vi "BeeHarmonicRadar.vi"(1 "Sampling Period":u32=10, 2 "Encoder Velocity Configuration":T1={"Right Encoder Rate to Velocity"=1.0, "Left Encoder Rate to Velocity"=1.0}, 3 "Reckoned Position FIFO Name":string="Position", 4 "Yaw RT FIFO":string="Yaw", 5 "Initial Values":T7, 6 "Encoder Dev Refs":T6={"RightEncoderDevRef"={"DevStatus"={"status"=FALSE, "code"=0, "source"=""}, "EncoderIndex"=enum."Invalid", "CounterIndex"=enum."Invalid", "DistancePerCount"=1.0, "Decoding Type"=enum."4x"}, "LeftEncoderDevRef"={"DevStatus"={"status"=FALSE, "code"=0, "source"=""}, "EncoderIndex"=enum."Invalid", "CounterIndex"=enum."Invalid", "DistancePerCount"=1.0, "Decoding Type"=enum."4x"}}) -> ()   [LabVIEW 2016]
uses:
  <vilib>/Rock Robotics/WPI/Encoder/WPI_EncoderDevRef.ctl
  <vilib>/Rock Robotics/SystemInterfaces/Encoder/FPGA_EncoderIdx.ctl
  <vilib>/Rock Robotics/SystemInterfaces/Counter/FPGA_CounterCtrSystemIndex.ctl
  <vilib>/Rock Robotics/WPI/Encoder/WPI_EncoderType.ctl
  <vilib>/Platform/TimedLoop/XDataNode/timing_clust.ctl
  <vilib>/Platform/TimedLoop/XDataNode/nitl_modes.ctl
  <vilib>/Platform/TimedLoop/XDataNode/wakeup.ctl
  <vilib>/platform/TimedLoop/XDataNode/XDataNode.xnode
  <vilib>/Platform/TimedLoop/XDataNode/XDNodeRunTimeDep.lvlib
panel:
  out "Y Trap + Gyro":dbl
  out "X Trap + Gyro":dbl
  in  "Reset":bool
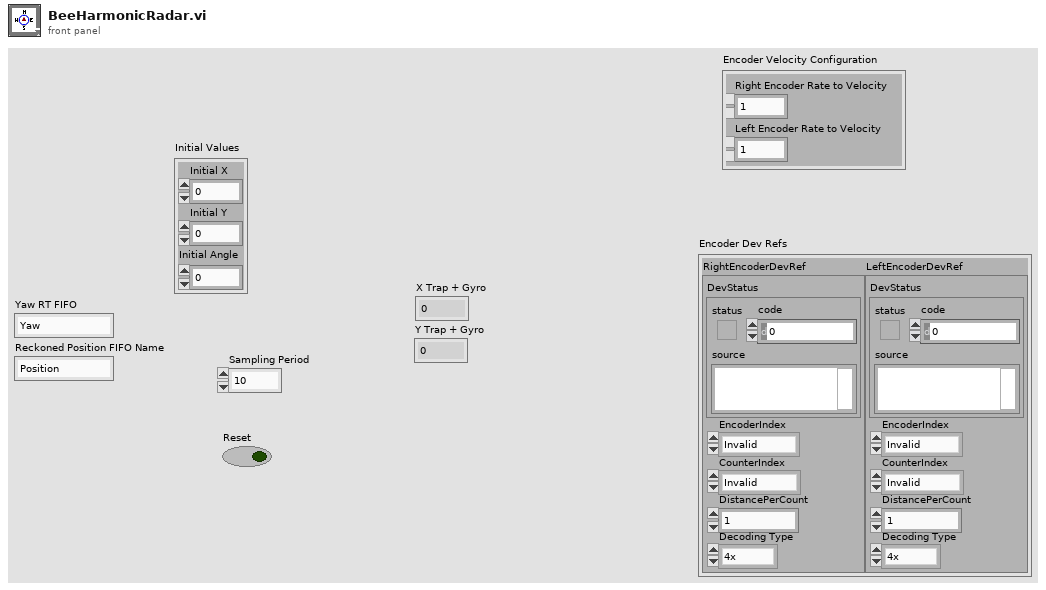
[diagram p1: front panel]
types:
  T1 = cluster{"Right Encoder Rate to Velocity":dbl, "Left Encoder Rate to Velocity":dbl}
  T2 = typedef "WPI_EncoderDevRef.ctl" = cluster{"DevStatus":errorcluster, "EncoderIndex":T3, "CounterIndex":T4, "DistancePerCount":dbl, "Decoding Type":T5}
  T3 = typedef "FPGA_EncoderIdx.ctl" = enum8{"Enc 0", "Enc 1", "Enc 2", "Enc 3", "Enc 4", "Enc 5", "Enc 6", "Enc 7", "Invalid"}
  T4 = typedef "FPGA_CounterCtrSystemIndex.ctl" = enum8{"Ctr 0", "Ctr 1", "Ctr 2", "Ctr 3", "Ctr 4", "Ctr 5", "Ctr 6", "Ctr 7", "Invalid"}
  T5 = typedef "WPI_EncoderType.ctl" = enum16{"1x", "2x", "4x"}
  T6 = cluster{"RightEncoderDevRef":T2, "LeftEncoderDevRef":T2}
  T7 = cluster{"Initial X":dbl, "Initial Y":dbl, "Initial Angle":dbl}
  T8 = typedef "XDNodeRunTimeDep.lvlib/timing_clust.ctl" = cluster{"Expected End [f-1]":u64, "Actual End [f-1]":u64, "Finished Late? [f-1]":bool, "Expected End [i-1]":u64, "Actual End [i-1]":u64, "Finished Late? [i-1]":bool, "Expected Start [i]":u64, "Actual Start [i]":u64, "Expected Start [f]":u64, "Actual Start [f]":u64, "Source Name":string, "Structure Name":string, "Period":i64, "Deadline":i64, "Offset":i64, "Start":i64, "Priority":i32, "Timeout":i32, "Mode":T9, "Wakeup Reason":T10, "Error":errorcluster, "Source Type":string, "Secondary Source Type":string, "Global End Time":u64, "Global Start Time":u64, "Frame Duration":u64, "Iteration Duration":u64, "Assigned CPU":i32, "I/O Scan Engine Mode":u32}
  T9 = typedef "XDNodeRunTimeDep.lvlib/nitl_modes.ctl" = enum32{"No Change", "Process missed periods, maintain original phase", "Discard missed periods, maintain original phase", "Process missed periods, ignore original phase", "Discard missed periods, ignore original phase"}
  T10 = typedef "XDNodeRunTimeDep.lvlib/wakeup.ctl" = enum32{"Normal", "Aborted", "Asynchronous wakeup", "Timing source error", "Timed loop error", "Timeout"}
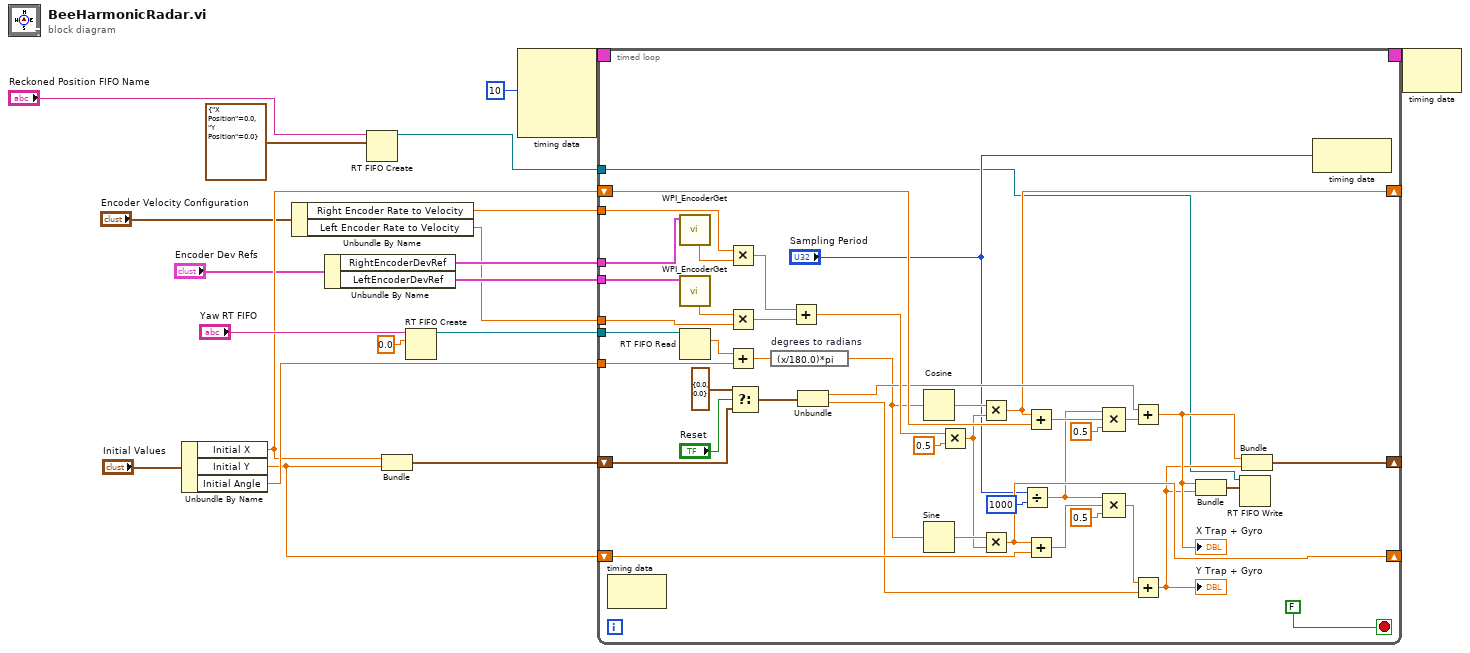
[diagram p0: block diagram]
diagram:
  n1 = Unbundle By Name("Initial Values") -> ("Initial X"=w7:dbl, "Initial Y"=w8:dbl, "Initial Angle"=w9:dbl)
  n2 = Unbundle By Name("Encoder Velocity Configuration") -> ("Right Encoder Rate to Velocity"=w2:dbl, "Left Encoder Rate to Velocity"=w1:dbl)
  n3 = Unbundle By Name("Encoder Dev Refs") -> ("RightEncoderDevRef"=w5:T2, "LeftEncoderDevRef"=w4:T2)
  n4 = RT FIFO Create(0:"Reckoned Position FIFO Name", 1:cluster{"X Position":dbl, "Y Position":dbl} {"X Position"=0.0, "Y Position"=0.0}) -> (8:w11:refnum<k33>)  [unwired: 6 in, 2 out]
  n5 = Bundle("Initial X"=w7, "Initial Y"=w8) -> (w20:cluster{"Initial X":dbl, "Initial Y":dbl})  [unwired: 1 in]
  n6 = RT FIFO Create(0:"Yaw RT FIFO", 1:0.0) -> (8:w16:refnum<k33>)  [unwired: 6 in, 2 out]
  n7 = node-c288(i64 10 ("Period")) -> (w19:T8)  [unwired: 3 in]
  n8 = timed-loop {
    tunnel: w9 -> [w62]
    shift-right: [w46] -> _
    shift-left: w8 -> [w60]
    shift-right: [w43] -> _
    shift-left: w7 -> [w59]
    shift-right: [w50] -> _
    shift-left: w20 -> [w32]
    timing: w19 -> [_]
    timing-out: [_] -> w18
    tunnel: w4 -> [w42]
    tunnel: w5 -> [w41]
    tunnel: w16 -> [w28]
    tunnel: w11 -> [w23]
    tunnel: w2 -> [w22]
    tunnel: w1 -> [w21]
    stop <- FALSE stop-if-true
    n9 = node-c288() -> ()  [unwired: 1 in, 1 out]
    n10 = call <vilib>:"WPI_EncoderGet.vi"("EncoderDevRef"=w41) -> ("Rate"=w30:dbl)  [unwired: 5 in, 5 out]
    n11 = call <vilib>:"WPI_EncoderGet.vi"("EncoderDevRef"=w42) -> ("Rate"=w29:dbl)  [unwired: 5 in, 5 out]
    n12 = RT FIFO Read(0:w28) -> (9:w27:dbl)  [unwired: 3 in, 4 out]
    n13 = Multiply(x=w22, y=w30) -> (x*y=w40:dbl)
    n14 = Multiply(x=w29, y=w21) -> (x*y=w39:dbl)
    n15 = Add(x=w27, y=w62) -> (x+y=w61:dbl)
    n16 = Select(t=cluster{"Initial X":dbl, "Initial Y":dbl} {"Initial X"=0.0, "Initial Y"=0.0}, s="Reset", f=w32) -> (s? t:f=w31:cluster{"Initial X":dbl, "Initial Y":dbl})
    n17 = expression code="(x/180.0)*pi" "degrees to radians"(w61) -> (w35:dbl)
    n18 = Add(x=w40, y=w39) -> (x+y=w58:dbl)
    n19 = Unbundle(w31) -> ("Initial X"=w49:dbl, "Initial Y"=w48:dbl)
    n20 = Cosine(x=w35) -> (cos(x)=w44:dbl)
    n21 = Sine(x=w35) -> (sin(x)=w47:dbl)
    n22 = Multiply(x=w58, y=0.5) -> (x*y=w45:dbl)
    n23 = Multiply(x=w44, y=w45) -> (x*y=w43:dbl)
    n24 = Multiply(x=w47, y=w45) -> (x*y=w46:dbl)
    n25 = Divide(x="Sampling Period", y=u32 1000) -> (x/y=w38:dbl)
    n26 = Add(x=w43, y=w59) -> (x+y=w55:dbl)
    n27 = Add(x=w46, y=w60) -> (x+y=w53:dbl)
    n28 = Compound Arithmetic op=MULTIPLY(w38, w55, 0.5 ("y")) -> (w52:dbl)
    n29 = Compound Arithmetic op=MULTIPLY(w38, w53, 0.5 ("y")) -> (w51:dbl)
    n30 = Add(x=w49, y=w52) -> (x+y=w26:dbl)
    "X Trap + Gyro" <- w26
    n31 = Add(x=w51, y=w48) -> (x+y=w25:dbl)
    "Y Trap + Gyro" <- w25
    n32 = Bundle(w26, w25) -> (w24:cluster{dbl, dbl})  [unwired: 1 in]
    n33 = RT FIFO Write(0:w23, 1:w24) -> ()  [unwired: 3 in, 4 out]
    n34 = Bundle(w26, w25) -> (w50:cluster{dbl, dbl})  [unwired: 1 in]
    n35 = node-c288("Sampling Period") -> ()  [unwired: 1 out]
  }
  n36 = node-c288(w18) -> ()  [unwired: 1 out]
